vi "RFConfig.vi"(8 "error in (no error)":errorcluster, 10 "接收参数设置":T2, 11 "发射参数设置":T1) -> (0 "error out":errorcluster)   [LabVIEW 2015]
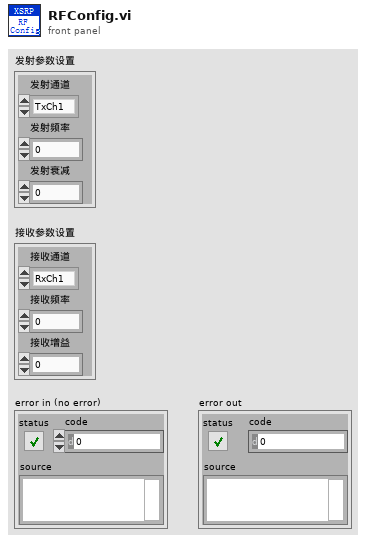
[diagram p1: front panel]
types:
  T1 = cluster{"发射通道":enum16{"TxCh1", "TxCh2"}, "发射频率":u32, "发射衰减":u8}
  T2 = cluster{"接收通道":enum16{"RxCh1", "RxCh2"}, "接收频率":u32, "接收增益":u8}
  T3 = cluster{"端口选择":string, "波特率":u32, "数据位":u16, "奇偶校验":u16, "停止位":u16, "流控":u16}
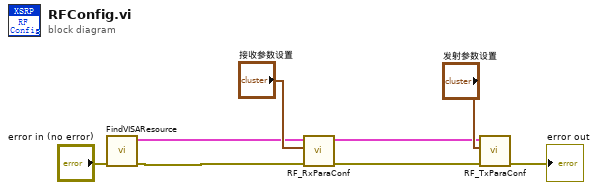
[diagram p0: block diagram]
diagram:
  n1 = call "FindVISAResource.vi"("error in (no error)"="error in (no error)") -> ("error out"=w1:errorcluster, "串口配置Out"=w2:T3)  [unwired: 9 in]
  n2 = call "RF_RxParaConf.vi"("error in"=w1, "DeviceConfiguare"="接收参数设置", "VISA IN"=w2) -> ("error out"=w3:errorcluster, "VISA OUT"=w5:T3)  [unwired: 7 in]
  n3 = call "RF_TxParaConf.vi"("error in"=w3, "硬件\n参数\n设置"="发射参数设置", "VISA IN"=w5) -> ("error OUT"=→"error out":errorcluster)  [unwired: 8 in]
